vi "PathSearch.vi"(0 "Path":dbl[][](array[numeric]), 5 "Reint":bool, 9 "Robot X (in)":dbl, 11 "Robot Y (in)":dbl, 12 "Search Window (s)":dbl=2.0, 13 "Look-Ahead Time (s)":dbl=0.25) -> (1 "Distance from Start (in)":dbl, 3 "Distance from End (in)":dbl, 4 "Feed Back Distance Error (in)":dbl, 6 "Feed Back Pointing Angle (deg)":dbl, 8 "Feed Forward Pointing Angle (deg)":dbl, 10 "Feed Forward Velocity (in/s)":dbl, 14 "Feed Forward Rotational Velocity (deg/s)":dbl, 15 "Robot Heading Goal (deg)":dbl)   [LabVIEW 2020]
doc: "This VI takes as input the robots current pose and the loaded autonomous path. The algorithm then efficiently searches the path and identifies the nearest point and the pursuit point. The the feed-forward heading, pointing direction, and velocity are output along with the error distance and and pointing direction required to return to the path. The distance along the path is also output. The Search Window can be specified in seconds - longer search windows are more robust to recovering from large deviations from the path but may cause the robot to \"jump\" ahead when following tight loops or turns. The Look-Ahead Time specifies the furthest ahead the pursuit point can be."
panel:
  out "Look-Ahead Point":i32
  out "Closest Point":i32
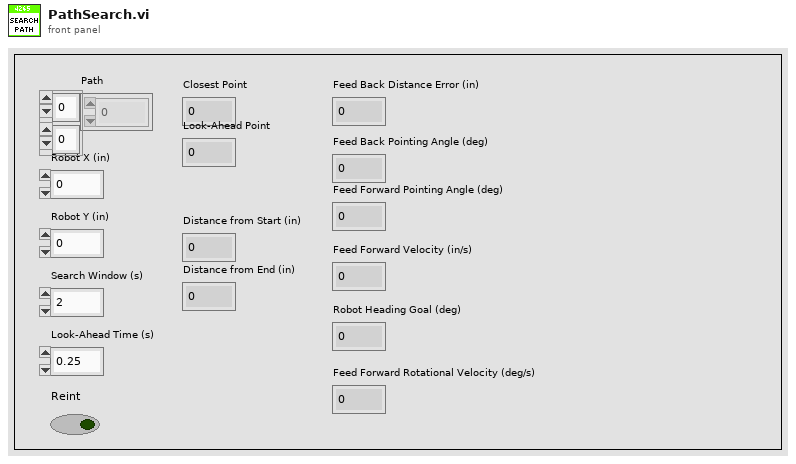
[diagram p1: front panel]
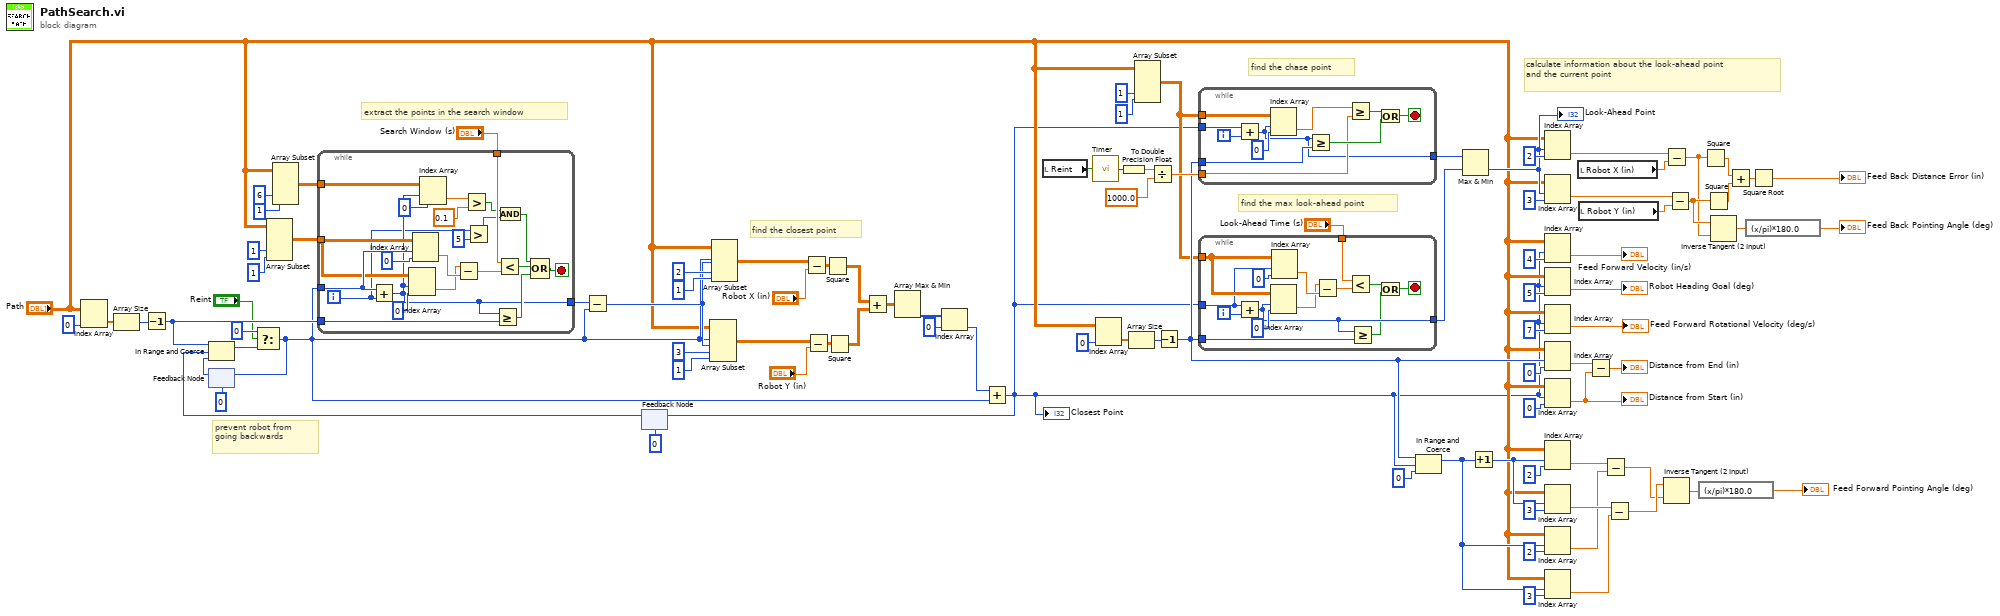
[diagram p0: block diagram]
diagram:
  # "find the chase point"
  # "find the max look-ahead point"
  # "calculate information about the look-ahead point\nand the current point"
  # "prevent robot from \ngoing backwards"
  # "find the closest point"
  # "extract the points in the search window"
  n1 = Index Array(array="Path", index (col)=0 ("disabled index (col)")) -> (element=w57:dbl[])  [unwired: 1 in]
  n2 = Array Size(array=w57) -> (size(s)=w58:i32)
  n3 = Decrement(x=w58) -> (x-1=w54:i32)
  n4 = feedback #1(0) -> (w55:i32)
  n5 = Array Subset(array="Path", index (col)=1 ("index"), length (col)=1 ("length")) -> (w78:dbl[][])  [unwired: 2 in]
  n6 = Array Subset(array="Path", index (col)=6 ("index"), length (col)=1 ("length")) -> (w5:dbl[][])  [unwired: 2 in]
  n7 = feedback #2(0) -> (w53:i32)
  n8 = In Range and Coerce(upper limit=w54, x=w53, lower limit=w55) -> (coerced(x)=w36:i32)  [unwired: 1 out]
  n9 = Select(t=0, s="Reint", f=w36) -> (s? t:f=w35:i32)
  n10 = feedback-in #1(w35) -> ()
  n11 = while {
    tunnel: w35 -> [w116]
    tunnel: w78 -> [w106]
    tunnel: "Search Window (s)" -> [w111]
    tunnel: [w101] -> w76
    tunnel: w54 -> [w107]
    tunnel: w5 -> [w105]
    i -> [w99]
    stop <- w109 stop-if-true
    # "Search window"
    n12 = Add(x=w116, y=w99) -> (x+y=w101:i32)
    n13 = Index Array(array=w106, index (row)=w101, index (col)=0 ("disabled index (col)")) -> (element=w113:dbl)
    n14 = Index Array(array=w106, index (row)=w116, index (col)=0 ("disabled index (col)")) -> (element=w114:dbl)
    n15 = Index Array(array=w105, index (row)=w101, index (col)=0 ("disabled index (col)")) -> (element=w104:dbl)
    n16 = Subtract(x=w113, y=w114) -> (x-y=w112:dbl)
    n17 = Greater?(x=w104, y=0.1) -> (0:w96:bool)
    n18 = Greater?(x=w99, y=5) -> (0:w100:bool)
    n19 = Greater Or Equal?(x=w101, y=w107) -> (x >= y?=w108:bool)
    n20 = Less?(x=w111, y=w112) -> (x < y?=w110:bool)
    n21 = And(x=w96, y=w100) -> (x .and. y?=w97:bool)
    n22 = Compound Arithmetic op=OR(w97, w110, w108) -> (w109:bool)
  }
  n23 = Subtract(x=w76, y=w35) -> (x-y=w75:i32)
  n24 = Array Subset(array="Path", index (row)=w35, length (row)=w75, index (col)=3 ("index"), length (col)=1 ("length")) -> (w87:dbl[][])
  n25 = Array Subset(array="Path", index (row)=w35, length (row)=w75, index (col)=2 ("index"), length (col)=1 ("length")) -> (w93:dbl[][])
  n26 = Subtract(x=w93, y="Robot X (in)") -> (x-y=w92:dbl[][])
  n27 = Subtract(x=w87, y="Robot Y (in)") -> (x-y=w88:dbl[][])
  n28 = Square(x=w92) -> (x^2=w85:dbl[][])
  n29 = Square(x=w88) -> (x^2=w84:dbl[][])
  n30 = Add(x=w85, y=w84) -> (x+y=w83:dbl[][])
  n31 = Array Max & Min(array=w83) -> (min index (indices)=w82:i32[])  [unwired: 3 out]
  n32 = Index Array(array=w82, index=0) -> (element=w74:i32)
  n33 = Add(x=w74, y=w35) -> (x+y=w2:i32)
  "Closest Point" <- w2
  n34 = feedback-in #2(w2) -> ()
  n35 = local read "Reint"() -> (w17:bool)
  n36 = call "Timer.vi"("Reset Timer"=w17) -> ("Time (ms)"=w16:u32)
  n37 = Index Array(array="Path", index (col)=0 ("disabled index (col)")) -> (element=w48:dbl[])  [unwired: 1 in]
  n38 = To Double Precision Float(number=w16) -> (double precision float=w14:dbl)
  n39 = Array Size(array=w48) -> (size(s)=w42:i32)
  n40 = Array Subset(array="Path", index (col)=1 ("index"), length (col)=1 ("length")) -> (w11:dbl[][])  [unwired: 2 in]
  n41 = Divide(x=w14, y=1000.0) -> (x/y=w13:dbl)
  n42 = Decrement(x=w42) -> (x-1=w12:i32)
  n43 = while {
    tunnel: w2 -> [w125]
    tunnel: w11 -> [w126]
    tunnel: w13 -> [w119]
    tunnel: w12 -> [w121]
    tunnel: [w118] -> w10
    i -> [w128]
    stop <- w123 stop-if-true
    # "Search window"
    n44 = Add(x=w125, y=w128) -> (x+y=w118:i32)
    n45 = Index Array(array=w126, index (row)=w118, index (col)=0 ("disabled index (col)")) -> (element=w120:dbl)
    n46 = Greater Or Equal?(x=w118, y=w121) -> (x >= y?=w122:bool)
    n47 = Greater Or Equal?(x=w120, y=w119) -> (x >= y?=w124:bool)
    n48 = Or(x=w124, y=w122) -> (x .or. y?=w123:bool)
  }
  n49 = while {
    tunnel: w2 -> [w139]
    tunnel: w11 -> [w140]
    tunnel: "Look-Ahead Time (s)" -> [w134]
    tunnel: [w133] -> w9
    tunnel: w12 -> [w129]
    i -> [w142]
    stop <- w131 stop-if-true
    # "Search window"
    n50 = Add(x=w139, y=w142) -> (x+y=w133:i32)
    n51 = Index Array(array=w140, index (row)=w133, index (col)=0 ("disabled index (col)")) -> (element=w136:dbl)
    n52 = Index Array(array=w140, index (row)=w139, index (col)=0 ("disabled index (col)")) -> (element=w137:dbl)
    n53 = Subtract(x=w136, y=w137) -> (x-y=w135:dbl)
    n54 = Less?(x=w134, y=w135) -> (x < y?=w132:bool)
    n55 = Greater Or Equal?(x=w133, y=w129) -> (x >= y?=w130:bool)
    n56 = Or(x=w132, y=w130) -> (x .or. y?=w131:bool)
  }
  n57 = In Range and Coerce(upper limit=w12, x=w2, lower limit=0) -> (coerced(x)=w20:i32)  [unwired: 1 out]
  n58 = Max & Min(x=w10, y=w9) -> (min(x,y)=w8:i32)  [unwired: 1 out]
  "Look-Ahead Point" <- w8
  n59 = Increment(x=w20) -> (x+1=w29:i32)
  n60 = Index Array(array="Path", index (row)=w8, index (col)=2 ("disabled index (col)")) -> (element=w71:dbl)
  n61 = Index Array(array="Path", index (row)=w8, index (col)=3 ("disabled index (col)")) -> (element=w69:dbl)
  n62 = Index Array(array="Path", index (row)=w2, index (col)=4 ("disabled index (col)")) -> (element=→"Feed Forward Velocity (in/s)":dbl)
  n63 = Index Array(array="Path", index (row)=w2, index (col)=5 ("disabled index (col)")) -> (element=→"Robot Heading Goal (deg)":dbl)
  n64 = Index Array(array="Path", index (row)=w2, index (col)=7 ("disabled index (col)")) -> (element=→"Feed Forward Rotational Velocity (deg/s)":dbl)
  n65 = Index Array(array="Path", index (row)=w12, index (col)=0 ("disabled index (row)")) -> (element=w39:dbl)
  n66 = Index Array(array="Path", index (row)=w2, index (col)=0 ("disabled index (col)")) -> (element=w37:dbl)
  "Distance from Start (in)" <- w37
  n67 = Index Array(array="Path", index (row)=w29, index (col)=2 ("disabled index (col)")) -> (element=w27:dbl)
  n68 = Index Array(array="Path", index (row)=w29, index (col)=3) -> (element=w28:dbl)
  n69 = Index Array(array="Path", index (row)=w20, index (col)=2) -> (element=w24:dbl)
  n70 = Index Array(array="Path", index (row)=w20, index (col)=3) -> (element=w23:dbl)
  n71 = local read "Robot X (in)"() -> (w70:dbl)
  n72 = local read "Robot Y (in)"() -> (w68:dbl)
  n73 = Subtract(x=w39, y=w37) -> (x-y=→"Distance from End (in)":dbl)
  n74 = Subtract(x=w27, y=w24) -> (x-y=w22:dbl)
  n75 = Subtract(x=w28, y=w23) -> (x-y=w31:dbl)
  n76 = Subtract(x=w71, y=w70) -> (x-y=w62:dbl)
  n77 = Inverse Tangent (2 Input)(1:w22, 2:w31) -> (0:w19:dbl)
  n78 = Subtract(x=w69, y=w68) -> (x-y=w63:dbl)
  n79 = expression code="(x/pi)*180.0"(w19) -> (→"Feed Forward Pointing Angle (deg)":dbl)
  n80 = Square(x=w62) -> (x^2=w66:dbl)
  n81 = Square(x=w63) -> (x^2=w67:dbl)
  n82 = Inverse Tangent (2 Input)(1:w62, 2:w63) -> (0:w61:dbl)
  n83 = Add(x=w66, y=w67) -> (x+y=w65:dbl)
  n84 = expression code="(x/pi)*180.0"(w61) -> (→"Feed Back Pointing Angle (deg)":dbl)
  n85 = Square Root(x=w65) -> (sqrt(x)=→"Feed Back Distance Error (in)":dbl)
